vi "LogiLAB.vi"() -> ()   [LabVIEW 2013]
uses:
  <vilib>/LabVIEW Interface for Arduino/Type Defs/Connection Type.ctl
  <vilib>/LabVIEW Interface for Arduino/Type Defs/Board Type.ctl
  <vilib>/Waveform/DWDTOps.llb/DWDT Analog to Digital.vi
  <vilib>/LabVIEW Interface for Arduino/LabVIEW Interface for Arduino.lvlib
panel:
  in  "Connection Type (USB/Serial)":T1
  in  "Bytes Per Packet (15)":u32=15
  in  "Baud Rate (115200)":u32=115200
  in  "VISA resource":refnum<visa-resource-name>
  in  "On/Off":bool
  in  "Digital Output Number":T2(radio)
  out "Digital Waveform Graph":digitalwaveform(graph)
  in  "Analog Output Number":enum32{"1", " 2", " 3", " 4", " 5", " 6"}(radio)
  out "Waveform Graph":dynamicdata(graph)
  # "LogiLab | By Ali Can oçal & Fouad Asil | supervisor : Assist. Prof. Dr. Murat AKSOY |2016"
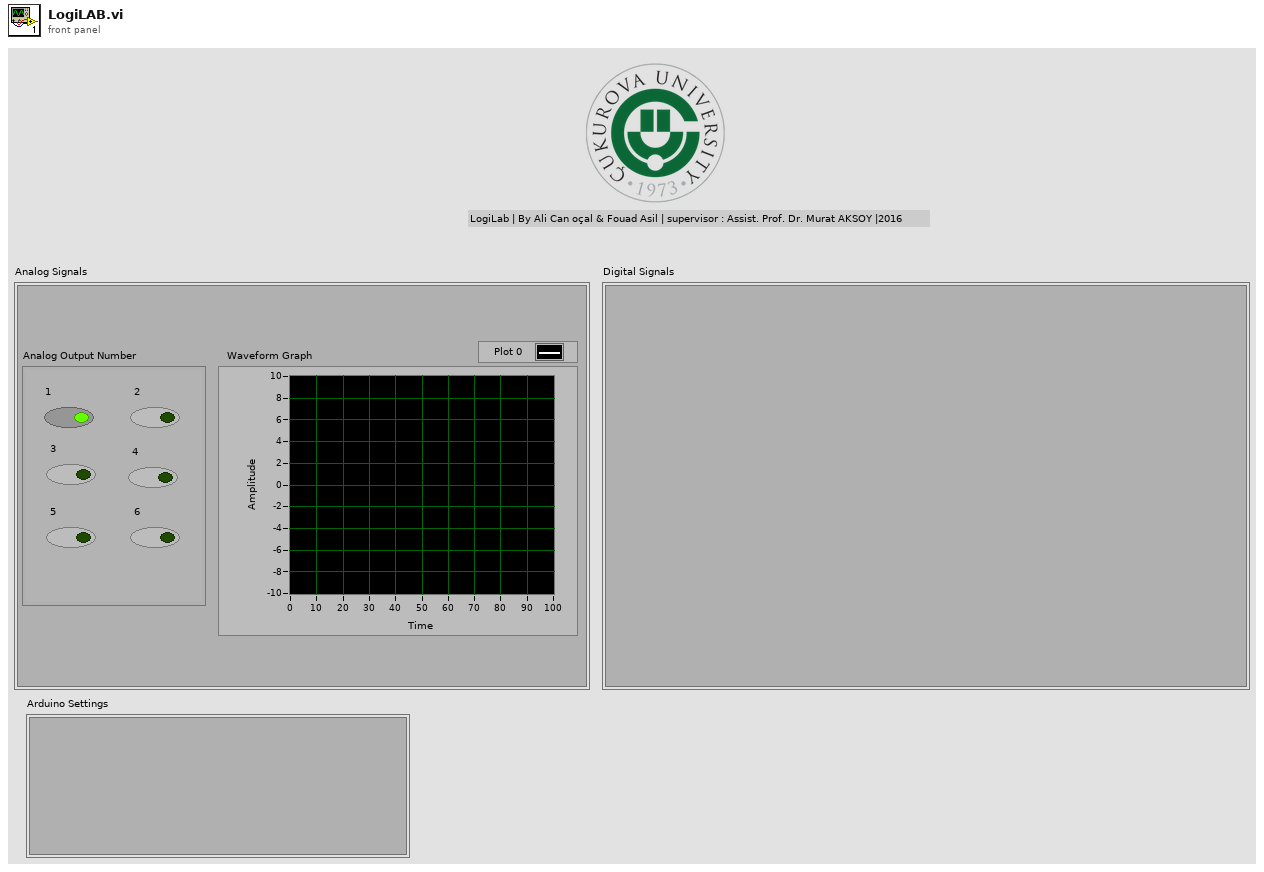
[diagram p1: front panel]
types:
  T1 = typedef "LabVIEW Interface for Arduino.lvlib/Connection Type.ctl" = enum8{"USB / Serial", "XBEE", "BlueSmirf (Bluetooth)"}
  T2 = enum32{"1", " 2", " 3", " 4", " 5", " 6", " 7", " 8"}
  T3 = typedef "LabVIEW Interface for Arduino.lvlib/Board Type.ctl" = enum16{"Uno", "Dimuelanove w/Atmega 328", "Mega 2560"}
  T4 = typedef "LabVIEW Interface for Arduino.lvlib/Arduino Resource.ctl" = cluster{"VISA resource":refnum<visa-resource-name>, "Board Type":T3, "Connection Type":enum8{"USB / Serial"}, "Bytes Per Packet (15)":u8}
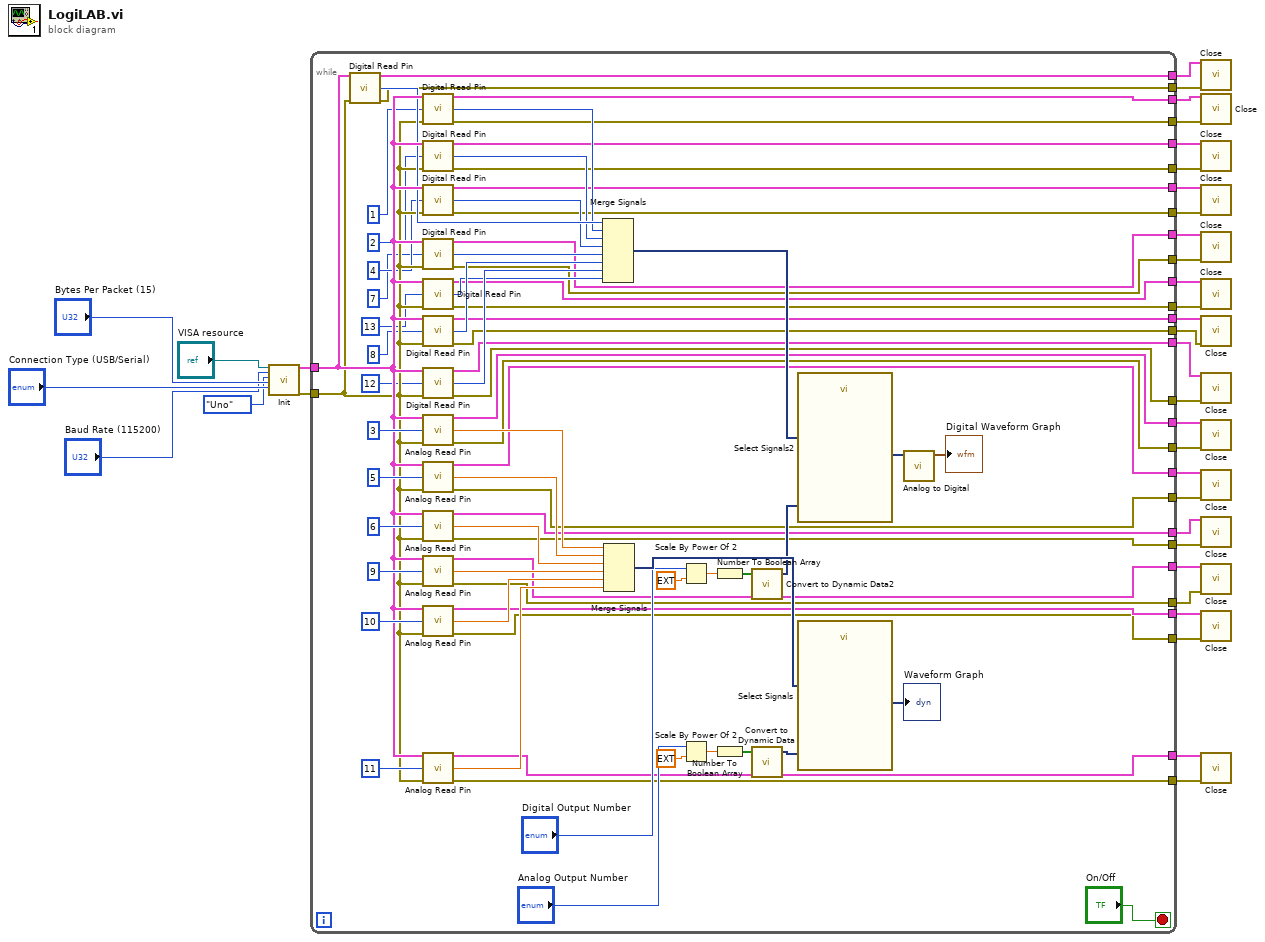
[diagram p0: block diagram]
diagram:
  n1 = call <vilib>:"Init.vi"("VISA resource"="VISA resource", "Baud Rate (115200)"="Baud Rate (115200)", "Board Type (Uno)"=Board_Type."Uno", "Bytes Per Packet (15)"="Bytes Per Packet (15)", "Connection Type (USB/Serial)"="Connection Type (USB/Serial)") -> ("Arduino Resource"=w30:T4, "error out"=w29:errorcluster)  [unwired: 13 in]
  n2 = while {
    tunnel: w30 -> [w88]
    tunnel: w29 -> [w57]
    tunnel: [w71] -> w28
    tunnel: [w70] -> w27
    tunnel: [w69] -> w26
    tunnel: [w68] -> w25
    tunnel: [w67] -> w24
    tunnel: [w66] -> w23
    tunnel: [w65] -> w22
    tunnel: [w64] -> w21
    tunnel: [w63] -> w20
    tunnel: [w62] -> w19
    tunnel: [w61] -> w18
    tunnel: [w60] -> w17
    tunnel: [w59] -> w16
    tunnel: [w58] -> w15
    tunnel: [w49] -> w14
    tunnel: [w48] -> w13
    tunnel: [w47] -> w12
    tunnel: [w46] -> w11
    tunnel: [w45] -> w10
    tunnel: [w44] -> w9
    tunnel: [w43] -> w8
    tunnel: [w42] -> w7
    tunnel: [w41] -> w6
    tunnel: [w40] -> w5
    tunnel: [w39] -> w4
    tunnel: [w38] -> w3
    tunnel: [w37] -> w2
    tunnel: [w36] -> w1
    stop <- "On/Off" stop-if-true
    n3 = call <vilib>:"Digital Read Pin.vi"("Arduino Resource"=w88, "error in"=w57) -> ("Arduino Resource"=w59:T4, "Value"=w87:u8, "error out"=w58:errorcluster)  [unwired: 11 in]
    n4 = call <vilib>:"Digital Read Pin.vi"("Arduino Resource"=w88, "Digital I/O Pin (0)"=u8 1, "error in"=w57) -> ("Arduino Resource"=w49:T4, "Value"=w86:u8, "error out"=w48:errorcluster)  [unwired: 10 in]
    n5 = call <vilib>:"Digital Read Pin.vi"("Arduino Resource"=w88, "Digital I/O Pin (0)"=u8 2, "error in"=w57) -> ("Arduino Resource"=w47:T4, "Value"=w85:u8, "error out"=w46:errorcluster)  [unwired: 10 in]
    n6 = call <vilib>:"Digital Read Pin.vi"("Arduino Resource"=w88, "Digital I/O Pin (0)"=u8 4, "error in"=w57) -> ("Arduino Resource"=w45:T4, "Value"=w84:u8, "error out"=w44:errorcluster)  [unwired: 10 in]
    n7 = call <vilib>:"Digital Read Pin.vi"("Arduino Resource"=w88, "Digital I/O Pin (0)"=u8 7, "error in"=w57) -> ("Arduino Resource"=w43:T4, "Value"=w83:u8, "error out"=w42:errorcluster)  [unwired: 10 in]
    n8 = call <vilib>:"Digital Read Pin.vi"("Arduino Resource"=w88, "Digital I/O Pin (0)"=u8 13, "error in"=w57) -> ("Arduino Resource"=w37:T4, "Value"=w80:u8, "error out"=w36:errorcluster)  [unwired: 10 in]
    n9 = call <vilib>:"Digital Read Pin.vi"("Arduino Resource"=w88, "Digital I/O Pin (0)"=u8 8, "error in"=w57) -> ("Arduino Resource"=w41:T4, "Value"=w82:u8, "error out"=w40:errorcluster)  [unwired: 10 in]
    n10 = call <vilib>:"Digital Read Pin.vi"("Arduino Resource"=w88, "Digital I/O Pin (0)"=u8 12, "error in"=w57) -> ("Arduino Resource"=w39:T4, "Value"=w81:u8, "error out"=w38:errorcluster)  [unwired: 10 in]
    n11 = call <vilib>:"Analog Read Pin.vi"("Arduino Resource"=w88, "Analog Input Pin (0)"=u8 3, "error in"=w57) -> ("Arduino Resource"=w71:T4, "Voltage"=w101:dbl, "error out"=w70:errorcluster)  [unwired: 10 in]
    n12 = call <vilib>:"Analog Read Pin.vi"("Arduino Resource"=w88, "Analog Input Pin (0)"=u8 5, "error in"=w57) -> ("Arduino Resource"=w69:T4, "Voltage"=w100:dbl, "error out"=w68:errorcluster)  [unwired: 10 in]
    n13 = call <vilib>:"Analog Read Pin.vi"("Arduino Resource"=w88, "Analog Input Pin (0)"=u8 6, "error in"=w57) -> ("Arduino Resource"=w67:T4, "Voltage"=w99:dbl, "error out"=w66:errorcluster)  [unwired: 10 in]
    n14 = call <vilib>:"Analog Read Pin.vi"("Arduino Resource"=w88, "Analog Input Pin (0)"=u8 9, "error in"=w57) -> ("Arduino Resource"=w65:T4, "Voltage"=w98:dbl, "error out"=w64:errorcluster)  [unwired: 10 in]
    n15 = call <vilib>:"Analog Read Pin.vi"("Arduino Resource"=w88, "Analog Input Pin (0)"=u8 10, "error in"=w57) -> ("Arduino Resource"=w63:T4, "Voltage"=w97:dbl, "error out"=w62:errorcluster)  [unwired: 10 in]
    n16 = call <vilib>:"Analog Read Pin.vi"("Arduino Resource"=w88, "Analog Input Pin (0)"=u8 11, "error in"=w57) -> ("Arduino Resource"=w61:T4, "Voltage"=w96:dbl, "error out"=w60:errorcluster)  [unwired: 10 in]
    n17 = Merge Signals(w87, w86, w85, w84, w83, w82, w81, w80) -> (w74:dynamicdata)
    n18 = Merge Signals(w101, w100, w99, w98, w97, w96) -> (w95:dynamicdata)
    n19 = Scale By Power Of 2(n="Digital Output Number", x=ext 1.0) -> (x*2^n=w77:ext)
    n20 = Scale By Power Of 2(n="Analog Output Number", x=ext 1.0) -> (x*2^n=w92:ext)
    n21 = Number To Boolean Array(number=w77) -> (Boolean array=w76:bool[])
    n22 = Number To Boolean Array(number=w92) -> (Boolean array=w91:bool[])
    n23 = call "Convert to Dynamic Data2"("Array"=w76) -> ("Dynamic Data Type"=w75:dynamicdata)  [unwired: 3 in]
    n24 = call "Convert to Dynamic Data"("Array"=w91) -> ("Dynamic Data Type"=w90:dynamicdata)  [unwired: 3 in]
    n25 = call "Select Signals2"("Selector Input"=w75, "Signals"=w74) -> ("Signal Out"=w73:dynamicdata)  [unwired: 8 in, 1 out]
    n26 = call "Select Signals"("Selector Input"=w90, "Signals"=w95) -> ("Signal Out"=→"Waveform Graph":dynamicdata)  [unwired: 8 in, 1 out]
    n27 = call-poly <vilib>:"Analog to Digital.vi"("analog waveform"=w73) -> ("digital waveform"=→"Digital Waveform Graph":digitalwaveform)  [unwired: 7 in, 3 out]
  }
  n28 = call <vilib>:"Close.vi"("Arduino Resource"=w16, "error in"=w15) -> ()  [unwired: 13 in, 1 out]
  n29 = call <vilib>:"Close.vi"("Arduino Resource"=w14, "error in"=w13) -> ()  [unwired: 13 in, 1 out]
  n30 = call <vilib>:"Close.vi"("Arduino Resource"=w12, "error in"=w11) -> ()  [unwired: 13 in, 1 out]
  n31 = call <vilib>:"Close.vi"("Arduino Resource"=w10, "error in"=w9) -> ()  [unwired: 13 in, 1 out]
  n32 = call <vilib>:"Close.vi"("Arduino Resource"=w8, "error in"=w7) -> ()  [unwired: 13 in, 1 out]
  n33 = call <vilib>:"Close.vi"("Arduino Resource"=w2, "error in"=w1) -> ()  [unwired: 13 in, 1 out]
  n34 = call <vilib>:"Close.vi"("Arduino Resource"=w6, "error in"=w5) -> ()  [unwired: 13 in, 1 out]
  n35 = call <vilib>:"Close.vi"("Arduino Resource"=w4, "error in"=w3) -> ()  [unwired: 13 in, 1 out]
  n36 = call <vilib>:"Close.vi"("Arduino Resource"=w28, "error in"=w27) -> ()  [unwired: 13 in, 1 out]
  n37 = call <vilib>:"Close.vi"("Arduino Resource"=w26, "error in"=w25) -> ()  [unwired: 13 in, 1 out]
  n38 = call <vilib>:"Close.vi"("Arduino Resource"=w24, "error in"=w23) -> ()  [unwired: 13 in, 1 out]
  n39 = call <vilib>:"Close.vi"("Arduino Resource"=w22, "error in"=w21) -> ()  [unwired: 13 in, 1 out]
  n40 = call <vilib>:"Close.vi"("Arduino Resource"=w20, "error in"=w19) -> ()  [unwired: 13 in, 1 out]
  n41 = call <vilib>:"Close.vi"("Arduino Resource"=w18, "error in"=w17) -> ()  [unwired: 13 in, 1 out]
